vi "Calculate Temperature Change.vi"(8 "error in (no error)":errorcluster) -> (0 "error out":errorcluster)   [LabVIEW 2018]
uses:
  Calculate Temperature Change-case.ctl
  <vilib>/addons/_JKI Toolkits/Caraya/classes/Test/Test.lvclass
  <vilib>/addons/_JKI Toolkits/Caraya/classes/Assert/Assert.lvclass
  Libraries/Thermal Chamber Response Simulator/Thermal Chamber Response Simulator.lvlib
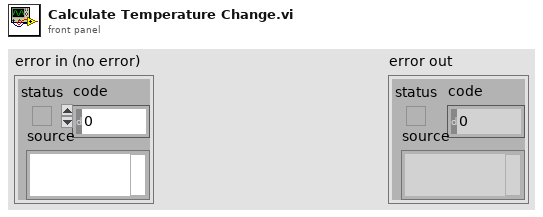
[diagram p1: front panel]
types:
  T1 = typedef "Calculate Temperature Change-case.ctl" = cluster{"test case ID":string, "Ramp Rate deg C/s":dbl, "Actual Temperature in deg C":dbl, "Time Interval (s)":dbl, "Shutdown":bool, "Required Temperature deg C":dbl, "Expected Actual Temperature":dbl}
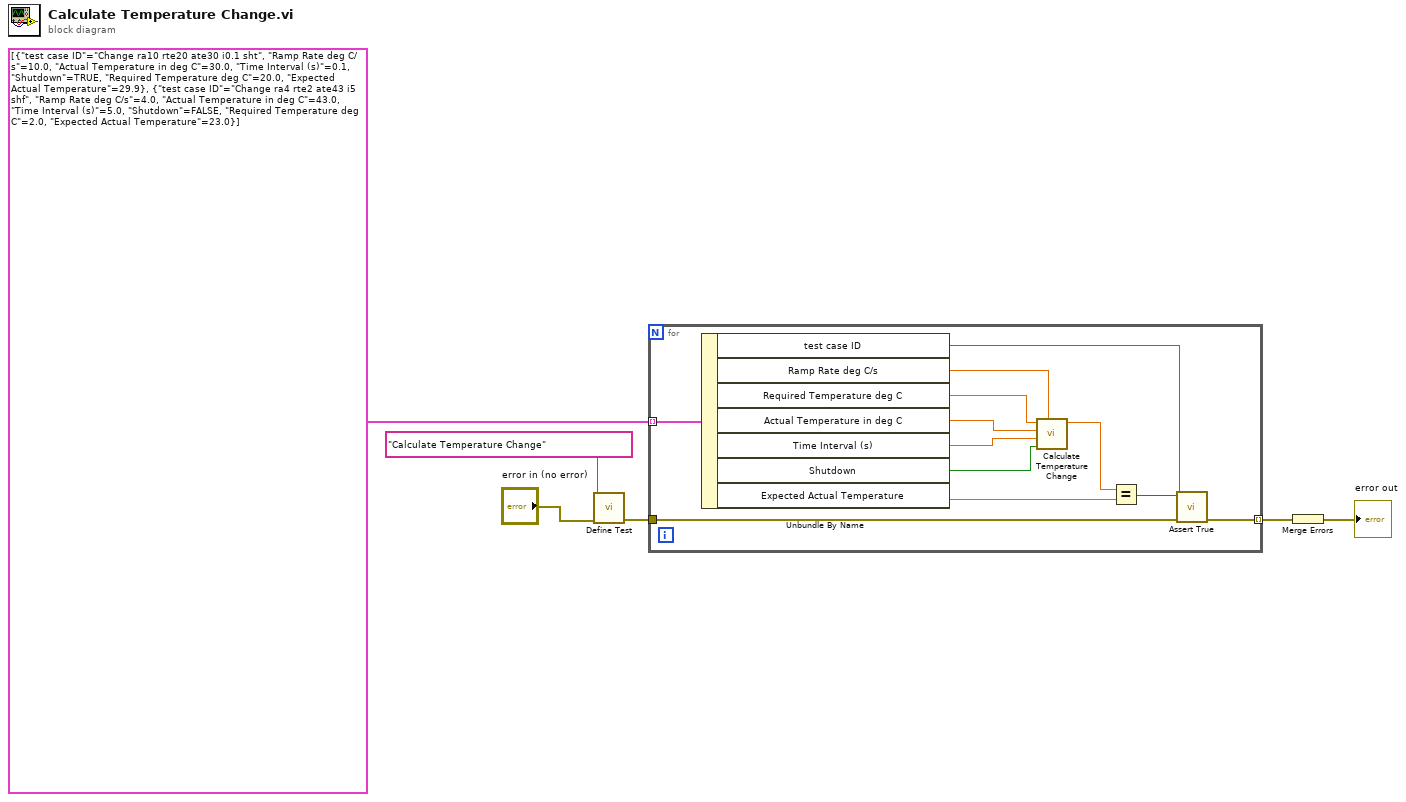
[diagram p0: block diagram]
diagram:
  n1 = call <vilib>:"Define Test.vi"("error in (no error)"="error in (no error)", "Label (VI Title)"="Calculate Temperature Change") -> ("error out"=w4:errorcluster)  [unwired: 9 in]
  n2 = for {
    tunnel: T1[] [{"test case ID"="Change ra10 rte20 ate30 i0.1 sht", "Ramp Rate deg C/s"=10.0, "Actual Temperature in deg C"=30.0, "Time Interval (s)"=0.1, "Shutdown"=TRUE, "Required Temperature deg C"=20.0, "Expected Actual Temperature"=29.9}, {"test case ID"="Change ra4 rte2 ate43 i5 shf", "Ramp Rate deg C/s"=4.0, "Actual Temperature in deg C"=43.0, "Time Interval (s)"=5.0, "Shutdown"=FALSE, "Required Temperature deg C"=2.0, "Expected Actual Temperature"=23.0}] -> [w18] mode=indexing
    tunnel: w4 -> [w8]
    tunnel: [w7] -> w3 mode=indexing
    n3 = Unbundle By Name(w18) -> ("test case ID"=w17:string, "Ramp Rate deg C/s"=w16:dbl, "Required Temperature deg C"=w15:dbl, "Actual Temperature in deg C"=w14:dbl, "Time Interval (s)"=w13:dbl, "Shutdown"=w12:bool, "Expected Actual Temperature"=w10:dbl)
    n4 = call "Calculate Temperature Change.vi"("Ramp Rate deg C/s"=w16, "Shutdown"=w12, "Time Interval (s)"=w13, "Actual Temperature in deg C"=w14, "Required Temperature deg C"=w15) -> ("Actual Temperature out"=w11:dbl)  [unwired: 6 in]
    n5 = Equal?(x=w11, y=w10) -> (x = y?=w9:bool)
    n6 = call <vilib>:"Assert True.vi"("Label"=w17, "error in (no error)"=w8, "True?"=w9) -> ("error out"=w7:errorcluster)  [unwired: 8 in]
  }
  n7 = Merge Errors(w3) -> (→"error out":errorcluster)
